vi "Teleop.vi"(10 "Match Info":T1={"Autonomous Elapsed Seconds"=0.0, "TeleOp Elapsed Seconds"=0.0, "Disabled Elapsed Seconds"=0.0, "Visited Autonomous"=FALSE, "Visited TeleOp"=FALSE, "Visited Disabled"=FALSE, "Autonomous Settings"={"Autonomous Style"=enum."Independent", "VI Refnum"=refnum}}, 11 "Call Context":T2) -> ()   [LabVIEW 2013]
doc: "This VI is called for each TeleOp packet received from the DS where the robot is not disabled. It is often used to read from the joysticks and update I/O or to update setpoints for timed control loops. It should complete and return within 20 milliseconds or it may miss DS packets."
uses:
  <vilib>/Rock Robotics/WPI/DriverStation/WPI_DriverStationDerivedRobotMode.ctl
  <vilib>/Rock Robotics/WPI/DriverStation/WPI_DriverStationMatch Info.ctl
  <vilib>/Rock Robotics/WPI/Relay/WPI_RelayValue.ctl
  <vilib>/Rock Robotics/WPI/Solenoid/WPI_SolenoidValue.ctl
  Robot Global Data.vi
  <vilib>/Rock Robotics/WPI/RobotDrive/WPI_RobotDriveArcadeDrive_Standard(NoSaturation).vi
  <vilib>/Rock Robotics/WPI/RobotDrive/WPI_RobotDriveGetSetRefNum.vi
  <vilib>/Rock Robotics/WPI/Joystick/WPI_JoystickGetSetRefNum.vi
  <vilib>/Rock Robotics/WPI/Solenoid/WPI_SolenoidSetEnum.vi
panel:
  out "Arm motor value":dbl
  in  "ball in grabber":bool
  out "Current value triggers":dbl
  in  "LEDs":bool
  out "Ball in grabber":bool
  in  "Use buttons?":bool
  out "Distance":dbl(slide) scale=0.0..254.0
  # "0.0098"
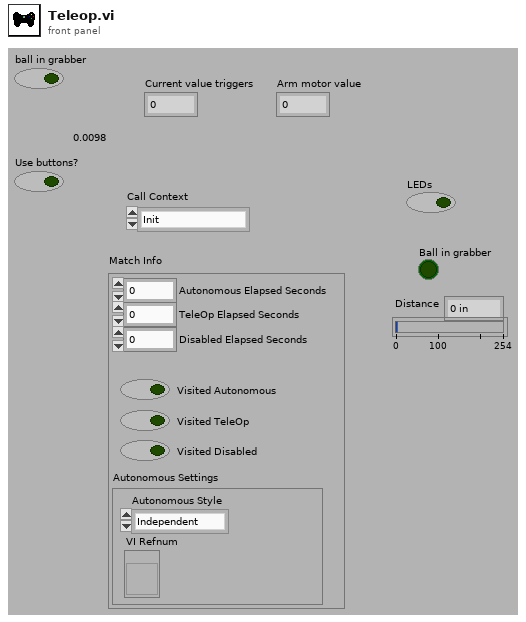
[diagram p1: front panel]
types:
  T1 = typedef "WPI_DriverStationMatch Info.ctl" = cluster{"Autonomous Elapsed Seconds":dbl, "TeleOp Elapsed Seconds":dbl, "Disabled Elapsed Seconds":dbl, "Visited Autonomous":bool, "Visited TeleOp":bool, "Visited Disabled":bool, "Autonomous Settings":cluster{"Autonomous Style":enum16{"Iterative", "Independent"}, "VI Refnum":refnum<vi>}}
  T2 = typedef "WPI_DriverStationDerivedRobotMode.ctl" = enum16{"Init", "Execute", "Stop"}
  T3 = typedef "WPI_CameraDevRef.ctl" = cluster{"Camera Address":string, "CameraStatus":errorcluster, "Acquire Image Notifier":refnum<notifier>}
  T4 = typedef "WPI_JoystickDevRef.ctl" = cluster{"Device":T5}
  T5 = typedef "WPI_JoystickDeviceEnum.ctl" = enum16{"USB 1", "USB 2", "USB 3", "USB 4", "Kinect 1", "Kinect 2"}
  T6 = typedef "WPI_JoystickButtonState.ctl" = cluster{"Button 1":bool, "Button 2":bool, "Button 3":bool, "Button 4":bool, "Button 5":bool, "Button 6":bool, "Button 7":bool, "Button 8":bool, "Button 9":bool, "Button 10":bool, "Button 11":bool, "Button 12":bool}
  T7 = cluster{"axis 1 (x)":dbl, "axis 2 (y)":dbl, "axis 3 (throttle)":dbl, "axis 4":dbl, "axis 5":dbl, "axis 6":dbl}
  T8 = typedef "WPI_RobotDriveDevRef.ctl" = cluster{"DevStatus":errorcluster, "Motors[]":T9[], "Square Inputs":bool, "Max Output":dbl, "Isochronous":bool}
  T9 = typedef "WPI_MotorControlDeviceRef.ctl" = cluster{"DeviceStatus":errorcluster, "Type":enum16{"PWM", "CAN"}, "PWM":cluster{"Digital Module":T10, "PWM Channel":T11, "DeadBand":T12}, "CAN":cluster{"Device Number":u8, "Control Mode":T13, "Semaphore":T14, "Max Vout":dbl}, "Invert":bool, "TransformRef":T15, "InvTransformRef":T15}
  T10 = typedef "FPGA_TypedefDigitalModule.ctl" = enum16{"Digital Module 1", "Digital Module 2"}
  T11 = typedef "FPGA_DIOPWMChannel.ctl" = enum8{"PWM 1", "PWM 2", "PWM 3", "PWM 4", "PWM 5", "PWM 6", "PWM 7", "PWM 8", "PWM 9", "PWM 10", "Invalid"}
  T12 = typedef "WPI_PWMDeadband.ctl" = cluster{"Name":string, "maxPositivePwm":i32, "minPositivePwm":i32, "centerPwm":i32, "maxNegativePwm":i32, "minNegativePwm":i32, "angularRange":u16}
  T13 = typedef "WPI_CANJaguar_ControlMode.ctl" = enum8{"Percent VBus", "Current", "Speed", "Position", "Voltage"}
  T14 = typedef "Semaphore RefNum" = refnum<k1>
  T15 = typedef "WPI_PWMTransform_ConPane.ctl" = refnum<vi>
  T16 = typedef "WPI_SolenoidDevRef.ctl" = cluster{"DevStatus":errorcluster, "Solenoid Module":T17, "Forward Solenoid Channel":T18, "Reverse Solenoid Channel":T18}
  T17 = typedef "FPGA_TypedefSolenoidModule.ctl" = enum16{"Solenoid Module 1", "Solenoid Module 2"}
  T18 = typedef "WPI_SolenoidChannel.ctl" = enum8{"Solenoid 1", "Solenoid 2", "Solenoid 3", "Solenoid 4", "Solenoid 5", "Solenoid 6", "Solenoid 7", "Solenoid 8", "Invalid"}
  T19 = typedef "WPI_SolenoidValue.ctl" = enum16{"Off", "On", "Forward", "Reverse"}
  T20 = typedef "WPI_AnalogChannelDevRef.ctl" = cluster{"DevStatus":errorcluster, "Analog Module":T21, "Analog Channel":T22}
  T21 = typedef "FPGA_TypedefAnalogModule.ctl" = enum16{"Analog Module 1", "Analog Module 2"}
  T22 = typedef "FPGA_AIChannel.ctl" = enum8{"AI 1", "AI 2", "AI 3", "AI 4", "AI 5", "AI 6", "AI 7", "AI 8", "Invalid"}
  T23 = typedef "WPI_RelayValue.ctl" = enum16{"Off", "On", "Forward", "Reverse"}
  T24 = typedef "WPI_RelayDevRef.ctl" = cluster{"DevStatus":errorcluster, "Relay Channel":T25, "Digital Module":T10, "Relay Direction":T26}
  T25 = typedef "FPGA_DIORelayChannel.ctl" = enum8{"Relay 1", "Relay 2", "Relay 3", "Relay 4", "Relay 5", "Relay 6", "Relay 7", "Relay 8", "Invalid"}
  T26 = typedef "WPI_RelayDirection.ctl" = enum16{"Both directions", "Forward only", "Reverse only"}
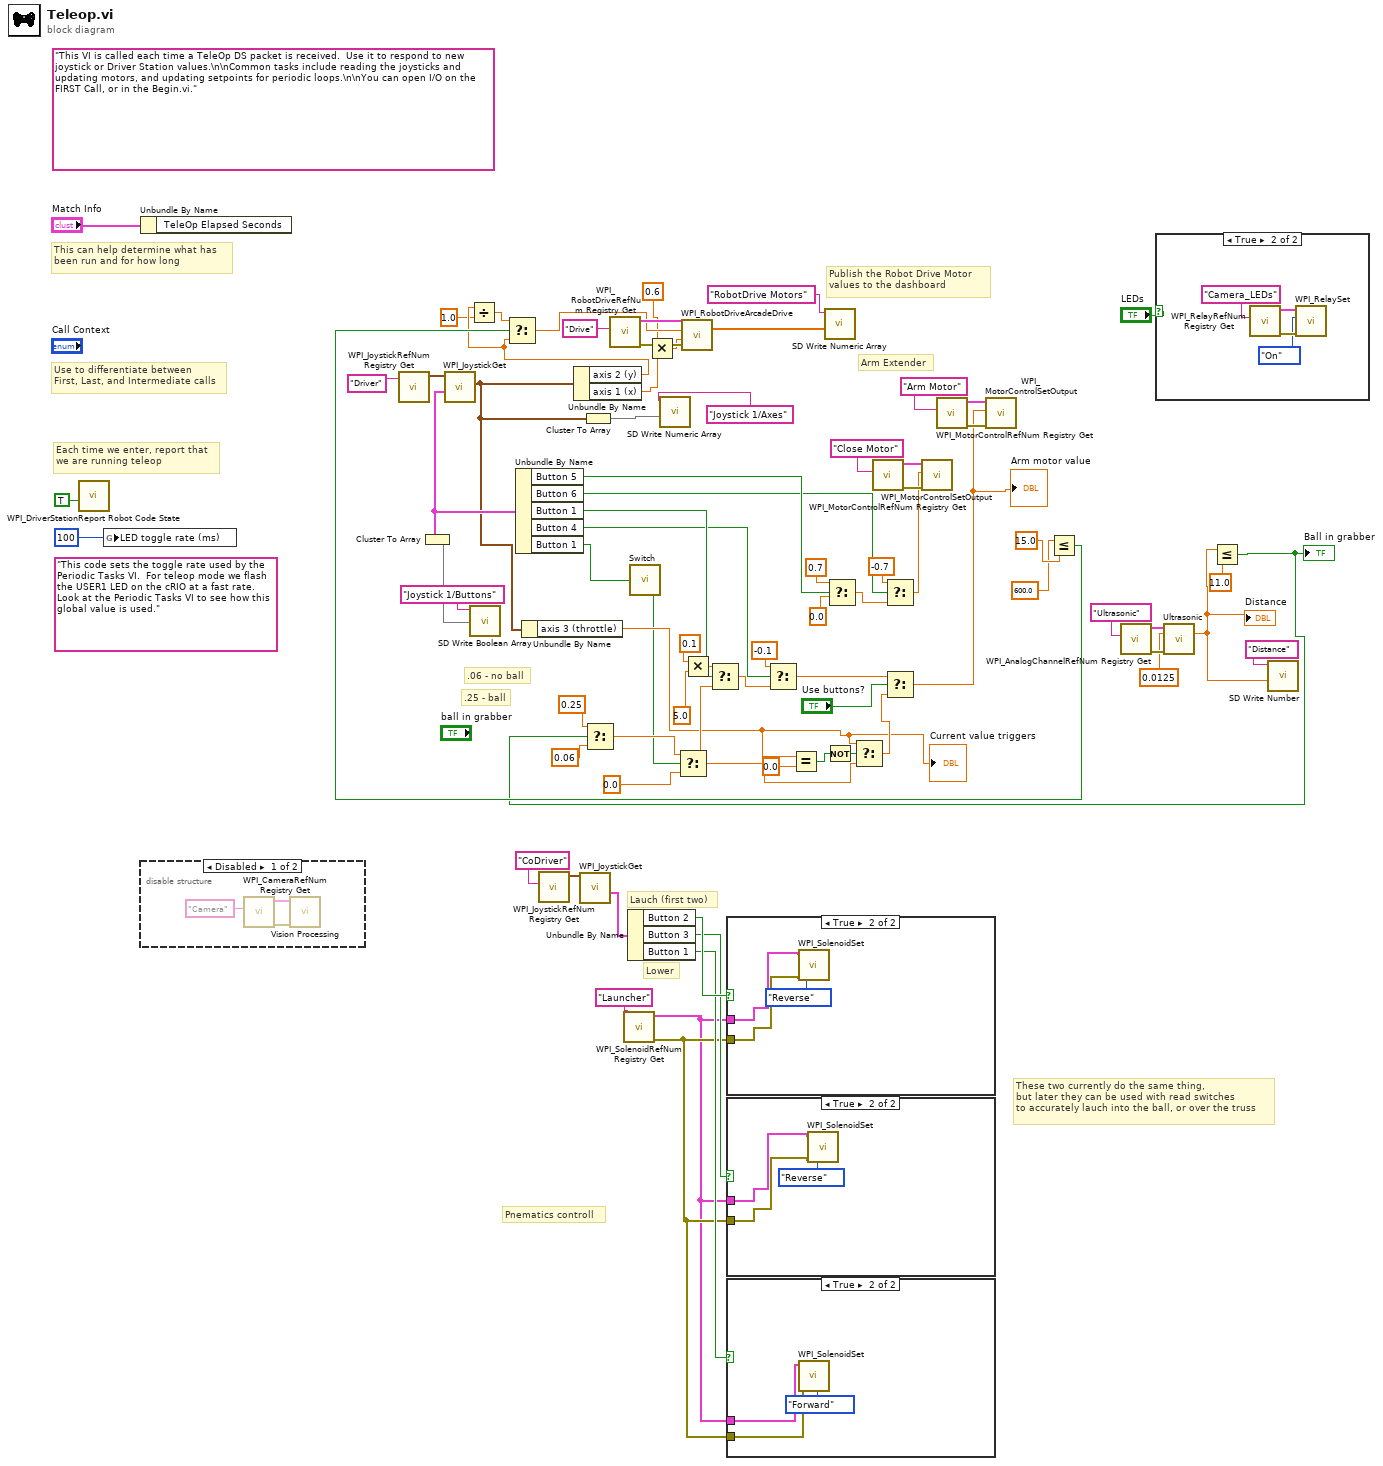
[diagram p0: block diagram]
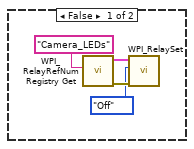
[diagram p3: hidden frame]
diagram:
  (unwired) "This code sets the toggle rate used by the Periodic Tasks VI.  For teleop mode we flash the USER1 LED on the cRIO at a fast rate.  Look at the Periodic Tasks VI to see how this global value is used."
  (unwired) "This VI is called each time a TeleOp DS packet is received.  Use it to respond to new joystick or Driver Station values.\n\nCommon tasks include reading the joysticks and updating motors, and updating setpoints for periodic loops.\n\nYou can open I/O on the FIRST Call, or in the Begin.vi."
  # ".25 - ball"
  # ".06 - no ball"
  # "Lauch (first two)"
  # "Lower"
  # "These two currently do the same thing,\nbut later they can be used with read switches\nto accurately lauch into the ball, or over the truss"
  # "Pnematics controll"
  # "Arm Extender"
  # "Publish the Robot Drive Motor\nvalues to the dashboard"
  # "Each time we enter, report that\nwe are running teleop"
  # "Use to differentiate between\nFirst, Last, and Intermediate calls"
  # "This can help determine what has\nbeen run and for how long"
  n1 = call <vilib>:"WPI_DriverStationReport Robot Code State.vi"("TeleOp"=TRUE ("Autonomous")) -> ()  [unwired: 10 in, 1 out]
  n2 = global write "Robot Global Data.vi" "LED toggle rate (ms)"(u32 100 ("LED ms toggle rate")) -> ()
  n3 = Unbundle By Name("Match Info") -> ()  [unwired: 1 out]
  n4 = disable-structure shown="Disabled" {
    frame Disabled {
      n5 = call <vilib>:"WPI_CameraRefNum Registry Get.vi"("refnum name"="Camera") -> ("error out"=w80:errorcluster, "CameraDevRef"=w81:T3)  [unwired: 9 in]
      n6 = call "Vision Processing.vi"("CameraDevRef"=w81, "error in"=w80) -> ()  [unwired: 25 in, 1 out]
    }
    frame Enabled {
    }
  }
  n7 = call <vilib>:"WPI_JoystickRefNum Registry Get.vi"("refnum name"="Driver") -> ("JoystickDevRef"=w74:T4)  [unwired: 1 in, 9 out]
  n8 = call <vilib>:"WPI_JoystickGet.vi"("JoystickDevRef"=w74) -> ("Buttons"=w67:T6, "Axes"=w35:T7)  [unwired: 1 in, 4 out]
  n9 = Cluster To Array(cluster=w67) -> (array=w73:bool[])
  n10 = call <vilib>:"SD Write Boolean Array.vi"("Boolean Array"=w73, "Name"="Joystick 1/Buttons") -> ()  [unwired: 8 in, 2 out]
  n11 = Unbundle By Name(w67) -> ("Button 5"=w38:bool, "Button 6"=w37:bool, "Button 1"=w49:bool, "Button 4"=w45:bool, "Button 1"=w3:bool)
  n12 = Unbundle By Name(w35) -> ("axis 3 (throttle)"=w19:dbl)
  "Current value triggers" <- w19
  n13 = call <vilib>:"WPI_JoystickRefNum Registry Get.vi"("refnum name"="CoDriver") -> ("JoystickDevRef"=w63:T4)  [unwired: 9 in, 1 out]
  n14 = Unbundle By Name(w35) -> ("axis 2 (y)"=w30:dbl, "axis 1 (x)"=w26:dbl)
  n15 = Divide(x=w30, y=1.0) -> (x/y=w31:dbl)
  n16 = call <vilib>:"WPI_JoystickGet.vi"("JoystickDevRef"=w63) -> ("Buttons"=w61:T6)  [unwired: 4 in, 2 out]
  n17 = Cluster To Array(cluster=w35) -> (array=w71:dbl[])
  n18 = call <vilib>:"WPI_RobotDriveRefNum Registry Get.vi"("refnum name"="Drive") -> ("error out"=w53:errorcluster, "RobotDriveDevRef"=w52:T8)  [unwired: 1 in, 8 out]
  n19 = call <vilib>:"WPI_SolenoidRefNum Registry Get.vi"("refnum name"="Launcher") -> ("error out"=w56:errorcluster, "SolenoidDevRef"=w55:T16)  [unwired: 9 in]
  n20 = Unbundle By Name(w61) -> ("Button 2"=w60:bool, "Button 3"=w59:bool, "Button 1"=w58:bool)
  n21 = call "Switch.vi"("In"=w3) -> ("out"=w2:bool)
  n22 = Multiply(x=0.6, y=w26) -> (x*y=w27:dbl)
  n23 = call <vilib>:"SD Write Numeric Array.vi"("Numeric Array"=w71, "Name"="Joystick 1/Axes") -> ()  [unwired: 8 in, 2 out]
  n24 = Multiply(x=0.1, y=5.0) -> (x*y=w48:dbl)
  n25 = case shown="True" w60 {
    tunnel: w55 -> [_ w85]
    tunnel: w56 -> [_ w84]
    frame False {
    }
    frame True {
      n26 = call-poly <vilib>:"WPI_SolenoidSet.vi"("error in (no error)"=w84, "Value"=WPI_SolenoidValue."Reverse", "SolenoidDevRef"=w85) -> ()  [unwired: 7 in, 2 out]
    }
  }
  n27 = case shown="True" w59 {
    tunnel: w55 -> [_ w88]
    tunnel: w56 -> [_ w87]
    frame False {
    }
    frame True {
      n28 = call-poly <vilib>:"WPI_SolenoidSet.vi"("error in (no error)"=w87, "Value"=WPI_SolenoidValue."Reverse", "SolenoidDevRef"=w88) -> ()  [unwired: 7 in, 2 out]
    }
  }
  n29 = case shown="True" w58 {
    tunnel: w56 -> [_ w90]
    tunnel: w55 -> [_ w91]
    frame False {
    }
    frame True {
      n30 = call-poly <vilib>:"WPI_SolenoidSet.vi"("error in (no error)"=w90, "Value"=WPI_SolenoidValue."Forward", "SolenoidDevRef"=w91) -> ()  [unwired: 7 in, 2 out]
    }
  }
  n31 = Equal?(x=w19, y=0.0) -> (x = y?=w17:bool)
  n32 = Not(x=w17) -> (.not. x?=w18:bool)
  n33 = Select(t=0.7, s=w38, f=0.0) -> (s? t:f=w40:dbl)
  n34 = call <vilib>:"WPI_MotorControlRefNum Registry Get.vi"("refnum name"="Close Motor") -> ("error out"=w66:errorcluster, "MotorControlDevRef"=w54:T9)  [unwired: 9 in]
  n35 = Select(t=-0.7, s=w37, f=w40) -> (s? t:f=w36:dbl)
  n36 = call <vilib>:"WPI_MotorControlSetOutput.vi"("error in (no error)"=w66, "Output"=w36, "MotorControlDevRef"=w54) -> ()  [unwired: 6 in, 3 out]
  n37 = call <vilib>:"WPI_MotorControlRefNum Registry Get.vi"("refnum name"="Arm Motor") -> ("error out"=w50:errorcluster, "MotorControlDevRef"=w68:T9)  [unwired: 9 in]
  n38 = Less Or Equal?(x=600.0, y=15.0 ("x")) -> (x <= y?=w32:bool)
  n39 = Select(t=w31, s=w32, f=w30) -> (s? t:f=w28:dbl)
  n40 = call-poly <vilib>:"WPI_RobotDriveArcadeDrive.vi"("error in (no error)"=w53, "Y axis value"=w27, "X axis value"=w28, "RobotDriveDevRef"=w52) -> ("Motor Values"=w51:dbl[])  [unwired: 5 in, 2 out]
  n41 = call <vilib>:"SD Write Numeric Array.vi"("Numeric Array"=w51, "Name"="RobotDrive Motors") -> ()  [unwired: 8 in, 2 out]
  n42 = call <vilib>:"WPI_AnalogChannelRefNum Registry Get.vi"("refnum name"="Ultrasonic") -> ("error out"=w12:errorcluster, "AIDeviceRef"=w11:T20)  [unwired: 9 in]
  n43 = case shown="True" "LEDs" {
    frame False {
      n44 = call <vilib>:"WPI_RelayRefNum Registry Get.vi"("refnum name"="Camera_LEDs") -> ("error out"=w94:errorcluster, "RelayDevRef"=w93:T24)  [unwired: 9 in]
      n45 = call <vilib>:"WPI_RelaySet.vi"("error in (no error)"=w94, "RelayValue"=WPI_RelayValue."Off", "RelayDevRef"=w93) -> ()  [unwired: 7 in, 2 out]
    }
    frame True {
      n46 = call <vilib>:"WPI_RelayRefNum Registry Get.vi"("refnum name"="Camera_LEDs") -> ("error out"=w98:errorcluster, "RelayDevRef"=w97:T24)  [unwired: 9 in]
      n47 = call <vilib>:"WPI_RelaySet.vi"("error in (no error)"=w98, "RelayValue"=WPI_RelayValue."On", "RelayDevRef"=w97) -> ()  [unwired: 7 in, 2 out]
    }
  }
  n48 = call "Ultrasonic.vi"("AIDeviceRef"=w11, "Scaling factor (Vcc/cm)"=0.0125, "error in (no error)"=w12) -> ("Distance"=w6:dbl)  [unwired: 10 in, 2 out]
  "Distance" <- w6
  n49 = Less Or Equal?(x=w6, y=11.0 ("x")) -> (x <= y?=w4:bool)
  "Ball in grabber" <- w4
  n50 = Select(t=0.25, s=w4, f=0.06) -> (s? t:f=w16:dbl)
  n51 = Select(t=w16, s=w2, f=0.0) -> (s? t:f=w21:dbl)
  n52 = Select(t=w48, s=w49, f=w21) -> (s? t:f=w43:dbl)
  n53 = Select(t=-0.1, s=w45, f=w43) -> (s? t:f=w34:dbl)
  n54 = Select(t=w19, s=w18, f=w21) -> (s? t:f=w20:dbl)
  n55 = Select(t=w34, s="Use buttons?", f=w20) -> (s? t:f=w1:dbl)
  "Arm motor value" <- w1
  n56 = call <vilib>:"WPI_MotorControlSetOutput.vi"("error in (no error)"=w50, "Output"=w1, "MotorControlDevRef"=w68) -> ()  [unwired: 6 in, 3 out]
  n57 = call <vilib>:"SD Write Number.vi"("Numeric"=w6, "Name"="Distance") -> ()  [unwired: 8 in, 2 out]
